vi "Test DAQmx Bus Analog Output.vi"() -> ()   [LabVIEW 2021]
uses:
  <vilib>/TSA/Omni-Bus/Omni-Bus/Omni_Bus.lvclass
  <vilib>/TSA/Omni-Bus/Omni-Bus/Support/Broad Types.ctl
  <vilib>/TSA/Abstract Data Classes/Abs_Types/Type/Abs_Type.lvclass/Abs_Type.ctl
  <vilib>/TSA/Omni-Bus/Omni-Bus/Omni_Bus.lvclass/Omni_Bus.ctl
  <vilib>/TSA/Omni-Bus/Omni-Bus/Support/Write/Write DBL.vi
  <vilib>/TSA/Omni-Bus/Omni-Bus/Support/FindVar.vi
  <vilib>/Utility/error.llb/Clear Errors.vi
  <vilib>/TSA/Omni-Bus/Omni-Bus/Properties/Read Var Map.vi
  <vilib>/TSA/Abstract Data Classes/Abs_Types/Type/Properties/Read Tag.vi
  Source/DAQmx-Bus.lvclass
  C:/Program Files (x86)/National Instruments/LabVIEW 2021/vi.lib/TSA/Omni-Bus/Omni-Bus/Bus Access/Bus_Access.lvclass
  <vilib>/TSA/Abstract Data Classes/Abs_Types/Double Float/Abs_Double Float.lvclass
  C:/Program Files (x86)/National Instruments/LabVIEW 2021/vi.lib/TSA/Abstract Data Classes/Abs_Types/Type/Abs_Type.lvclass
  <vilib>/TSA/Abstract Data Classes/Abs_Types/Value/Abs_Value.lvclass
  <vilib>/TSA/Omni-Bus/Omni-Bus/Support/Check For Read Only Error.vi
  <vilib>/TSA/Omni-Bus/Omni-Bus/Support/Incorrect Tag String Error.vi
  <vilib>/TSA/Abstract Data Classes/Abs_Types/Type/Abs_Type.lvclass
panel:
  in  "Slide":dbl(slide) scale=-5.0..5.0
  out "timed out?":bool
  in  "stop":bool
  in  "Combo Box":string(combo)
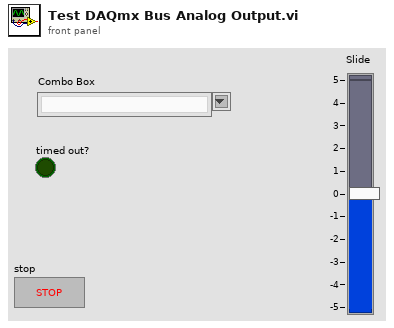
[diagram p1: front panel]
types:
  T1 = typedef "Omni_Bus.lvclass/Broad Types.ctl" = enum16{"All Tags", "NI Specific Type", "Boolean", "String", "Numeric", "Float", "Integer", "Collection", "All Value Types", "Non Value Types"}
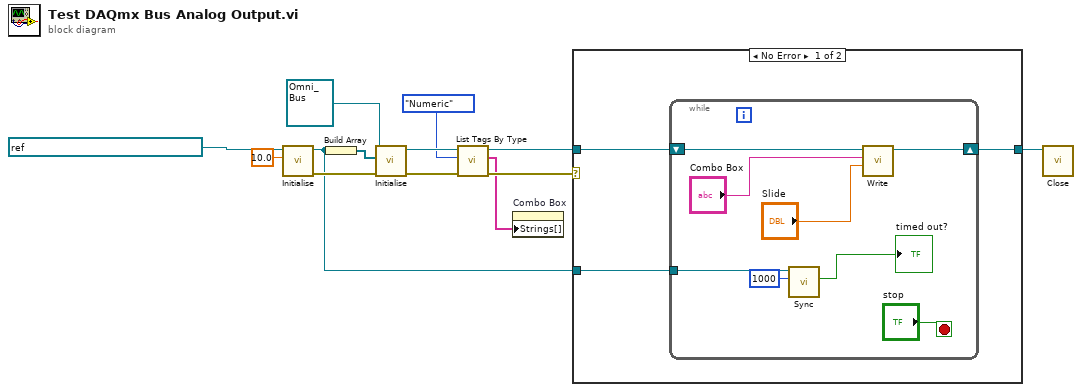
[diagram p0: block diagram]
diagram:
  n1 = call "Initialise.vi"("timeout (s)"=10.0 ("timeout"), "DAQmx Device"=refnum<k21> "MyVoltageOutTask_Ondemand") -> ("error out"=w9:errorcluster, "DAQmx-Bus out"=w1:refnum<class "DAQmx-Bus.lvclass">)  [unwired: 8 in]
  n2 = Build Array(w1) -> (w11:refnum<class "DAQmx-Bus.lvclass">[])
  n3 = call-dynamic "Initialise.vi"("error in (no error)"=w9, "Bus Access"=w11, "Var Bus in"=refnum<class "Omni_Bus.lvclass"> refnum) -> ("error out"=w6:errorcluster, "Var Bus out"=w7:refnum<class "Omni_Bus.lvclass">)  [unwired: 7 in]
  n4 = call <vilib>:"List Tags By Type.vi"("error in (no error)"=w6, "Broad Types"=Broad_Types."Numeric", "Var Bus in"=w7) -> ("error out"=w4:errorcluster, "Tags"=w3:string[], "Var Bus out"=w5:refnum<class "Omni_Bus.lvclass">)  [unwired: 5 in, 1 out]
  n5 = property on="Combo Box" class="CmbBox"("Strings[]"=w3) -> ()  [unwired: 2 in, 2 out]
  n6 = case shown="No Error" w4 {
    tunnel: [w16 w25] -> w8
    tunnel: w5 -> [w15 w25]
    tunnel: w1 -> [w14 _]
    frame No Error {
      n7 = while {
        shift-right: [w24] -> w16
        shift-left: w15 -> [w23]
        tunnel: w14 -> [w20]
        stop <- "stop" stop-if-true
        n8 = call-dynamic "Sync.vi"("timeout in ms (-1)"=1000, "DAQmx-Bus in"=w20) -> ("timed out?"=→"timed out?":bool)  [unwired: 7 in, 2 out]
        n9 = call-poly <vilib>:"Write.vi"("Numeric"="Slide", "Tag"="Combo Box", "Omni_Bus in"=w23) -> ("Omni_Bus out"=w24:refnum<class "Omni_Bus.lvclass">)  [unwired: 7 in, 1 out]
      }
    }
    frame Error {
    }
  }
  n10 = call-dynamic "Close.vi"("Data in"=w8) -> ()  [unwired: 9 in, 2 out]
